vi "GC EX Vacuum - Step 5.vi"(7 "Step":i32, 8 "error in":errorcluster, 9 "Test Results In":T8, 10 "Gas":T1, 11 "GC Configuration":T2) -> (0 "error out":errorcluster, 1 "Test Results Out":T8, 2 "Gas Out":T1 caption="Gas", 3 "GC Configuration Out":T2)   [LabVIEW 2015]
uses:
  Controls/Test Information.ctl
  Controls/Vacuum Test.ctl
  Controls/Test Timing.ctl
  Controls/Vaccum Thresholds.ctl
  Controls/Helium Test.ctl
  Controls/Helium Thresholds.ctl
  CAN Communication/Gas/Typedefs/Session Handle.ctl
  CAN Communication/Gas/Gas.lvclass
  Controls/Test Results.ctl
  Controls/Step Result.ctl
  CAN Communication/Gas/Typedefs/Valves.ctl
  SubVIs/Timing/Timing.lvlib
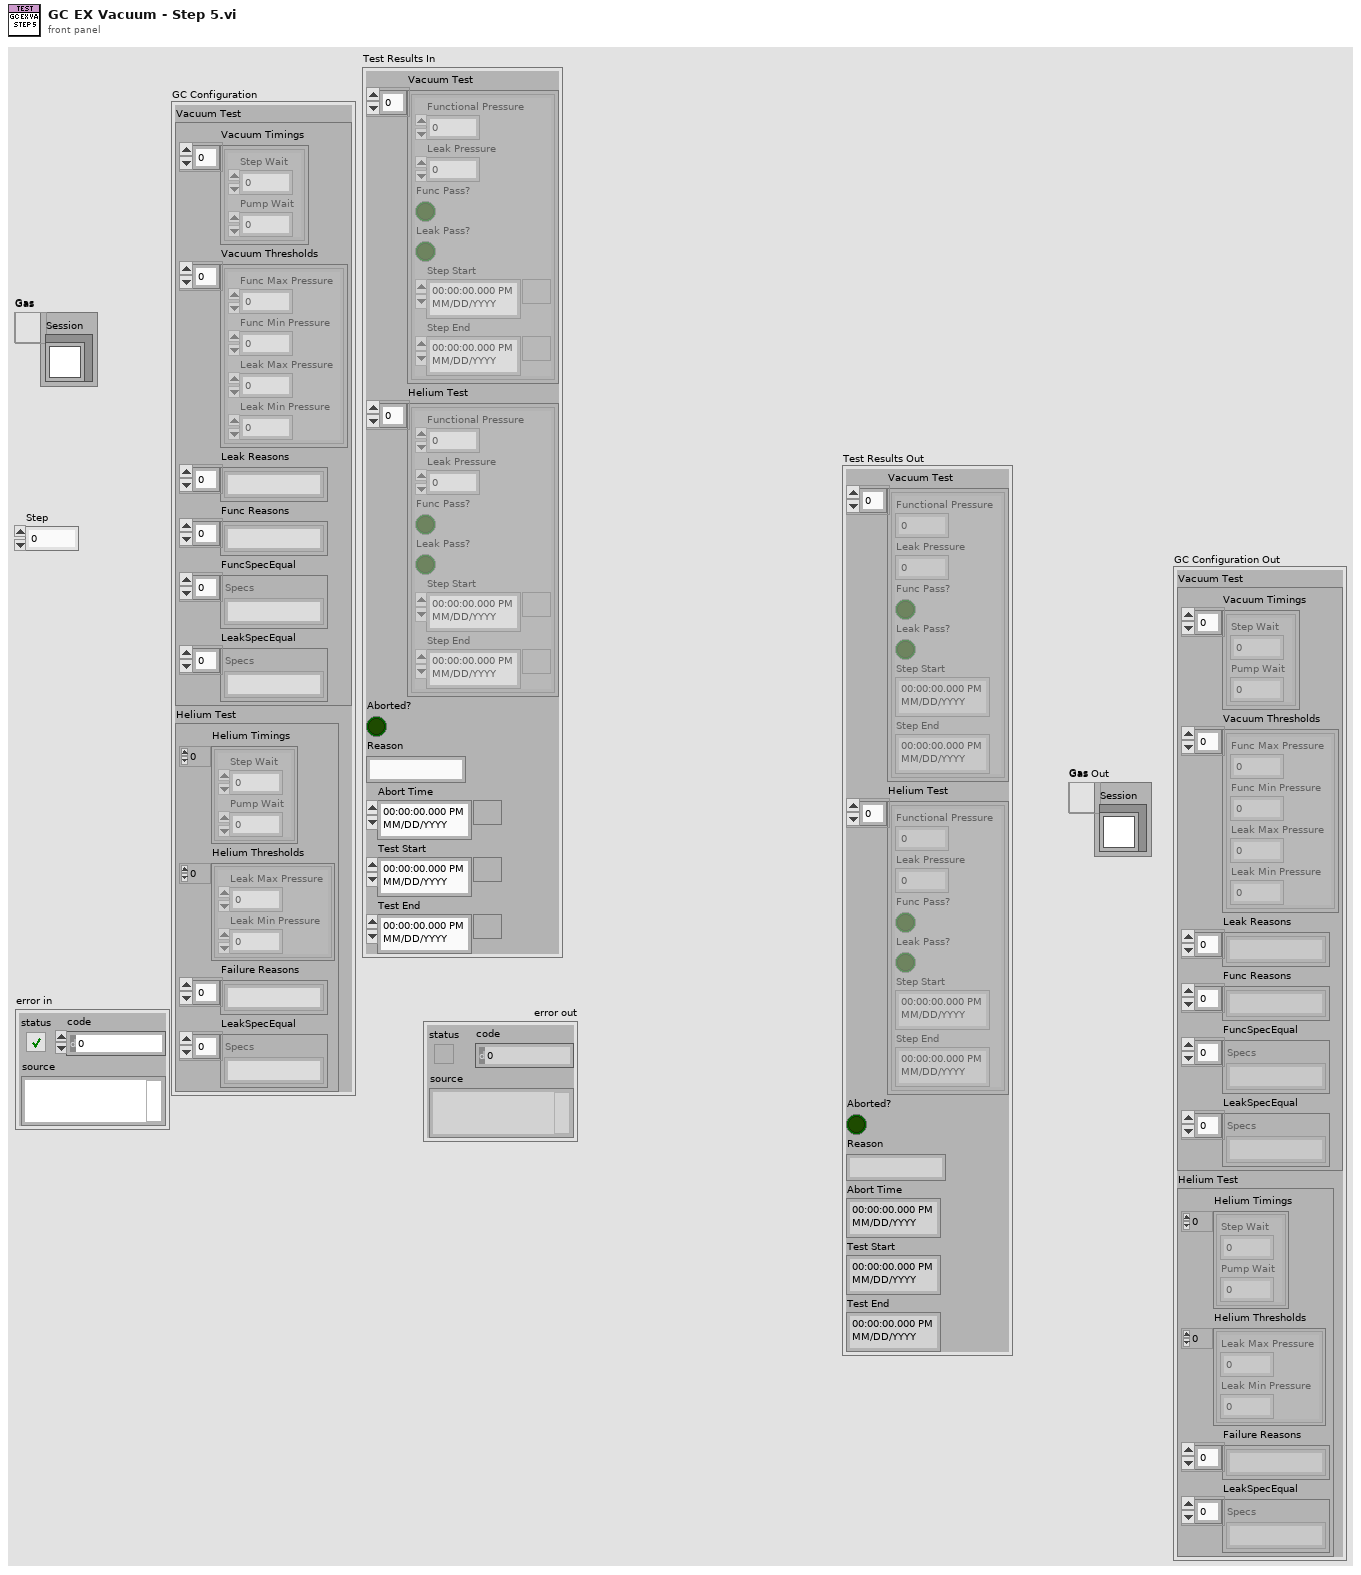
[diagram p1: front panel]
types:
  T1 = typedef "Gas.lvclass/Session Handle.ctl" = refnum<data-value>
  T2 = typedef "Test Information.ctl" = cluster{"Vacuum Test":T3, "Helium Test":T6}
  T3 = typedef "Vacuum Test.ctl" = cluster{"Vacuum Timings":T4[], "Vacuum Thresholds":T5[], "Leak Reasons":string[], "Func Reasons":string[], "FuncSpecEqual":string[], "LeakSpecEqual":string[]}
  T4 = typedef "Test Timing.ctl" = cluster{"Step Wait":dbl, "Pump Wait":dbl}
  T5 = typedef "Vaccum Thresholds.ctl" = cluster{"Func Max Pressure":dbl, "Func Min Pressure":dbl, "Leak Max Pressure":dbl, "Leak Min Pressure":dbl}
  T6 = typedef "Helium Test.ctl" = cluster{"Helium Timings":T4[], "Helium Thresholds":T7[], "Failure Reasons":string[], "LeakSpecEqual":string[]}
  T7 = typedef "Helium Thresholds.ctl" = cluster{"Leak Max Pressure":dbl, "Leak Min Pressure":dbl}
  T8 = typedef "Test Results.ctl" = cluster{"Vacuum Test":T9[], "Helium Test":T9[], "Aborted?":bool, "Reason":string, "Abort Time":timestamp, "Test Start":timestamp, "Test End":timestamp}
  T9 = typedef "Step Result.ctl" = cluster{"Functional Pressure":dbl, "Leak Pressure":dbl, "Func Pass?":bool, "Leak Pass?":bool, "Step Start":timestamp, "Step End":timestamp}
  T10 = typedef "Gas.lvclass/Valves.ctl" = u16
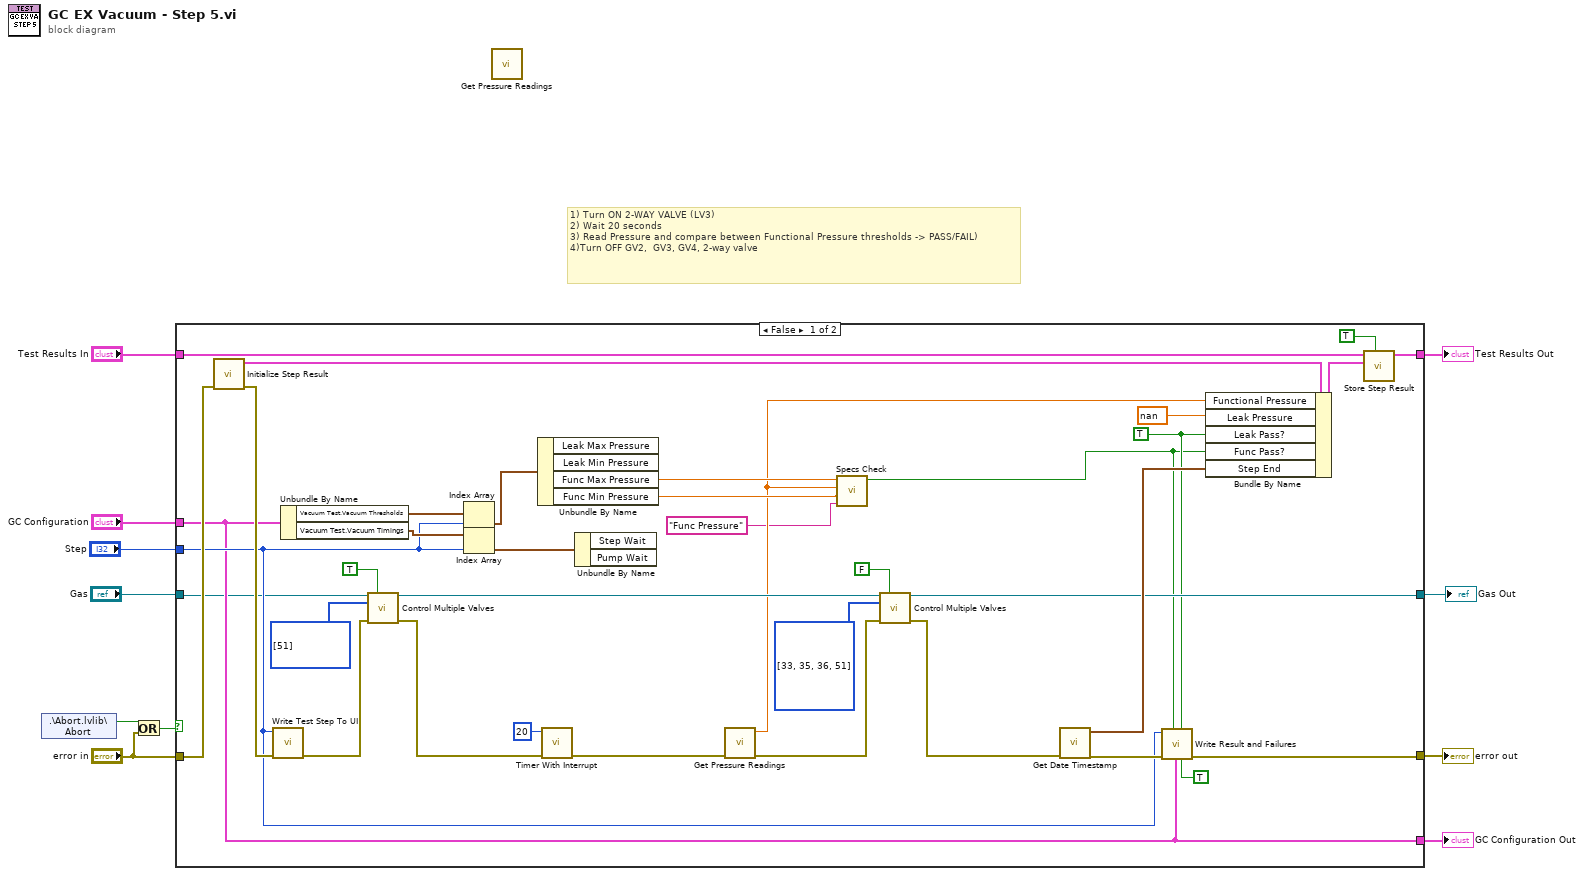
[diagram p0: block diagram]
diagram:
  # "1) Turn ON 2-WAY VALVE (LV3)\n2) Wait 20 seconds\n3) Read Pressure and compare between Functional Pressure thresholds -> PASS/FAIL)\n4)Turn OFF GV2,  GV3, GV4, 2-way valve"
  n1 = shared-variable ".\\Abort.lvlib\\Abort"() -> (w10:bool)  [unwired: 1 in, 1 out]
  n2 = Or(x=w10, y="error in") -> (x .or. y?=w9:bool)
  n3 = case shown="False" w9 {
    tunnel: "error in" -> [w48 w51]
    tunnel: "Test Results In" -> [w45 w52]
    tunnel: [w46 w52] -> w7
    tunnel: [w36 w51] -> w6
    tunnel: "GC Configuration" -> [w34 w50]
    tunnel: "Step" -> [w35 _]
    tunnel: [w34 w50] -> w3
    tunnel: [w25 w49] -> w1
    tunnel: "Gas" -> [w33 w49]
    frame False {
      w23 = T10[] [33, 35, 36, 51] items=["GV1"=33, "GV2"=34, "GV3"=35, "GV4"=36, "GV5"=37, "GV6"=38, "GV7"=39, "GV8"=40, "GV9"=41, "GV10"=42, "GV11"=43, "LV3"=51, "LV4"=52] ("Valves")
      w19 = TRUE ("Func Pass?")
      w32 = T10[] [51] items=["GV1"=33, "GV2"=34, "GV3"=35, "GV4"=36, "GV5"=37, "GV6"=38, "GV7"=39, "GV8"=40, "GV9"=41, "GV10"=42, "GV11"=43, "LV3"=51, "LV4"=52] ("Valves")
      n4 = call "Initialize Step Result.vi"("error in (no error)"=w48) -> ("error out"=w47:errorcluster, "New Step Result"=w44:T9)  [unwired: 8 in, 1 out]
      n5 = call "Write Test Step To UI.vi"("error in (no error)"=w47, "Step"=w35) -> ("error out"=w30:errorcluster)  [unwired: 9 in]
      n6 = Unbundle By Name(w34) -> ("Vacuum Test.Vacuum Thresholds"=w41:T5[], "Vacuum Test.Vacuum Timings"=w40:T4[])
      n7 = call "Control Multiple Valves.vi"("Session Handle in"=w33, "Energize?"=TRUE, "Valves"=w32, "error in (no error)"=w30) -> ("Session Handle out"=w26:T1, "error out"=w29:errorcluster)  [unwired: 8 in, 2 out]
      n8 = Index Array(array=w41, index=w35) -> (element=w38:T5)
      n9 = Index Array(array=w40, index=w35) -> (element=w39:T4)
      n10 = Unbundle By Name(w38) -> ("Func Max Pressure"=w15:dbl, "Func Min Pressure"=w14:dbl)  [unwired: 2 out]
      n11 = call "Timer With Interrupt.vi"("error in (no error)"=w29, "Wait (s)"=20) -> ("error out"=w27:errorcluster)  [unwired: 7 in, 2 out]
      n12 = Unbundle By Name(w39) -> ()  [unwired: 2 out]
      n13 = call "Get Pressure Readings.vi"("error in (no error)"=w27) -> ("error out"=w22:errorcluster, "NI-DAQ Pressure"=w13:dbl)  [unwired: 6 in, 3 out]
      n14 = call "Specs Check.vi"("parameter"="Func Pressure", "lower limit"=w14, "x"=w13, "upper limit"=w15) -> ("In Range?"=w16:bool)  [unwired: 6 in, 1 out]
      n15 = call "Control Multiple Valves.vi"("Session Handle in"=w26, "Energize?"=FALSE, "Valves"=w23, "error in (no error)"=w22) -> ("Session Handle out"=w25:T1, "error out"=w21:errorcluster)  [unwired: 8 in, 2 out]
      n16 = call "Get Date Timestamp.vi"("error in (no error)"=w21) -> ("error out"=w37:errorcluster, "current time"=w42:timestamp)  [unwired: 9 in]
      n17 = call "Write Result and Failures.vi"("Vacuum?"=TRUE, "Leak"=w19, "GC Configuration"=w34, "Func"=w16, "error in (no error)"=w37, "Step"=w35) -> ("error out"=w36:errorcluster)  [unwired: 5 in]
      n18 = Bundle By Name(cluster=w44, "Functional Pressure"=w13, "Leak Pressure"=nan ("Functional Pressure"), "Leak Pass?"=w19, "Func Pass?"=w16, "Step End"=w42) -> (w43:T9)
      n19 = call "Store Step Result.vi"("Vacuum?"=TRUE, "Step Result"=w43, "Test Results In"=w45) -> ("Test Results Out"=w46:T8)  [unwired: 8 in]
    }
    frame True {
    }
  }
  "error out" <- w6
  "Test Results Out" <- w7
  "GC Configuration Out" <- w3
  "Gas Out" <- w1
  n20 = call "Get Pressure Readings.vi"() -> ()  [unwired: 7 in, 5 out]
